vi "setTemperature.vi"(8 "error in (no error)":errorcluster, 10 "setTemperature":dbl, 11 "CameraNetworkController in":refnum<class "CameraNetworkController.lvclass">) -> (0 "error out":errorcluster, 3 "CameraNetworkController out":refnum<class "CameraNetworkController.lvclass">)   [LabVIEW 2011, in "Hardware.lvlib" / "HWControllers.lvlib" / "CameraNetworkController.lvclass"]
uses:
  CameraNetworkController.lvclass
  NetworkClient/NetworkServer.lvclass
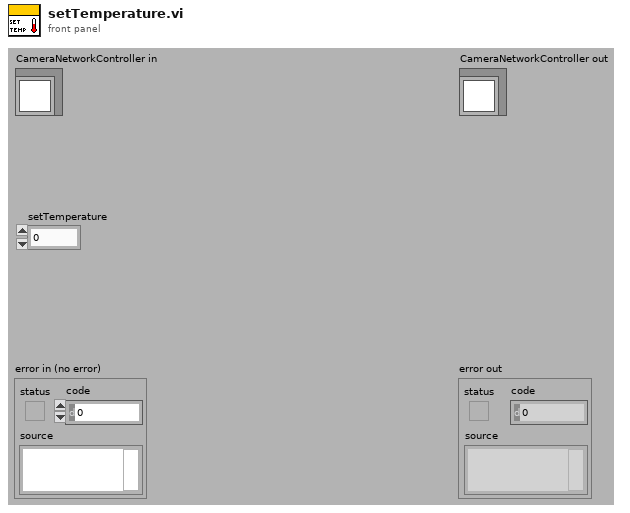
[diagram p1: front panel]
types:
  T1 = cluster{"Message":enum16{"Idle", "initialise", "configureAcquisition", "setTemperature", "getTemperature", "start", "stop", "sendImage", "close", "error", "ExitApp"}, "Data":variant}
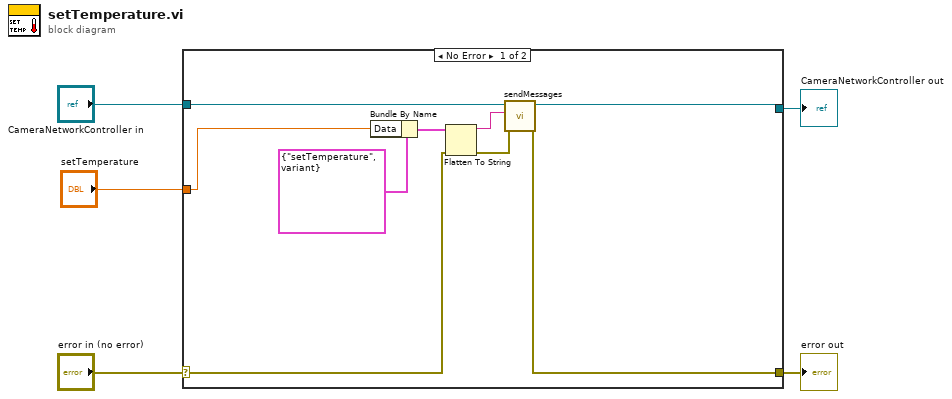
[diagram p0: block diagram]
diagram:
  n1 = case shown="No Error" "error in (no error)" {
    selector: "error in (no error)" -> [w6 w16]
    tunnel: [w8 w16] -> w4
    tunnel: [w9 w15] -> w2
    tunnel: "CameraNetworkController in" -> [w10 w15]
    tunnel: "setTemperature" -> [w7 _]
    frame No Error {
      n2 = Bundle By Name(cluster=T1 {"Message"=enum."setTemperature", "Data"=variant}, "Data"=w7) -> (w13:T1)
      n3 = Flatten To String(anything=w13, error in (no error)=w6) -> (data string=w11:string, error out=w12:errorcluster)  [unwired: 3 out]
      n4 = call "sendMessages.vi"("error in (no error)"=w12, "messageString"=w11, "NetworkClient in"=w10) -> ("error out"=w8:errorcluster, "NetworkClient out"=w9:refnum<class "CameraNetworkController.lvclass">)  [unwired: 7 in]
    }
    frame Error {
    }
  }
  "error out" <- w4
  "CameraNetworkController out" <- w2
